vi "Scatter2008.vi"   [LabVIEW 2013]
uses:
  <vilib>/Heliosphere Research LLC/Advanced Plotting Toolkit/Advanced Plotting Toolkit.lvlib
types:
  T1 = typedef "Advanced Plotting Toolkit.lvlib/PlotID.ctl" = i32
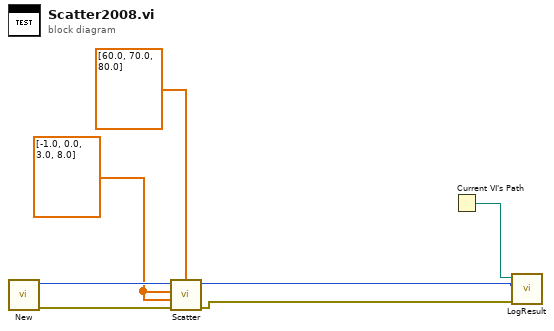
[diagram p0: block diagram]
diagram:
  w2 = dbl[] [-1.0, 0.0, 3.0, 8.0] ("X Data")
  n1 = call <vilib>:"New.vi"() -> ("error out"=w5:errorcluster, "Plot ID"=w6:T1)  [unwired: 10 in]
  n2 = call <vilib>:"Scatter.vi"("Areas"=dbl[] [60.0, 70.0, 80.0] ("X Data"), "error in (no error)"=w5, "Y Data"=w2, "X Data"=w2, "Plot ID"=w6) -> ("error out"=w3:errorcluster, "Plot ID Out"=w4:T1)  [unwired: 5 in]
  n3 = Current VI's Path() -> (path=w7:path)
  n4 = call "LogResult.vi"("Test Result"=w3, "Test Artifact"=w4, "VI Path"=w7) -> ()  [unwired: 9 in]
